vi "Pre Launch Init.vi"(11 "Study Actor in":refnum<class "Study Actor.lvclass">) -> (0 "error out":errorcluster, 3 "Study Actor out":refnum<class "Study Actor.lvclass">)   [LabVIEW 2023, in "HAL GOOP4.lvlib" / "Study Actor.lvlib" / "Study Actor.lvclass"]
doc: "Initializes the panel actor. Creates the Panel Helper.\n\n----\nPlease see the following web address for additional documentation and tutorial information:\nhttp://www.mooregoodideas.com/mgi-panel-manager/\n\nAuthor: Derek Trepanier\n\nCopyright (c) 2018, Moore Good Ideas, Inc.\n\nAll rights reserved.\n\nRedistribution and use in source and binary forms, with or without modification, are permitted provided that the following conditions are met:\n\n * Redistributions of source code must retain the above copyright notice, this list of conditions and the following disclaimer.\n * Redistributions in binary form must reproduce the above copyright notice, this list of conditions and the following disclaimer in the documentation and/or other materials provided with the distribution.\n * Neither the name of Moore Good Ideas, Inc. nor the names of its contributors may be used to endorse or promote products derived from this software without specific prior written permission.\n\nTHIS SOFTWARE IS PROVIDED BY THE COPYRIGHT HOLDERS AND CONTRIBUTORS \"AS IS\" AND ANY EXPRESS OR IMPLIED WARRANTIES, INCLUDING, BUT NOT LIMITED TO, THE IMPLIED WARRANTIES OF MERCHANTABILITY AND FITNESS FOR A PARTICULAR PURPOSE ARE DISCLAIMED. IN NO EVENT SHALL THE COPYRIGHT OWNER OR CONTRIBUTORS BE LIABLE FOR ANY DIRECT, INDIRECT, INCIDENTAL, SPECIAL, EXEMPLARY, OR CONSEQUENTIAL DAMAGES (INCLUDING, BUT NOT LIMITED TO, PROCUREMENT OF SUBSTITUTE GOODS OR SERVICES; LOSS OF USE, DATA, OR PROFITS; OR BUSINESS INTERRUPTION) HOWEVER CAUSED AND ON ANY THEORY OF LIABILITY, WHETHER IN CONTRACT, STRICT LIABILITY, OR TORT (INCLUDING NEGLIGENCE OR OTHERWISE) ARISING IN ANY WAY OUT OF THE USE OF THIS SOFTWARE, EVEN IF ADVISED OF THE POSSIBILITY OF SUCH DAMAGE."
uses:
  Study Actor.lvclass
  Study Actor.lvclass/Study Actor.ctl
  <vilib>/MGI/Panel Manager/Panel Actor/Panel Actor/Panel Actor.lvclass
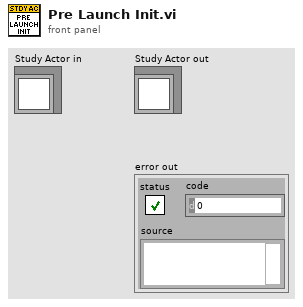
[diagram p1: front panel]
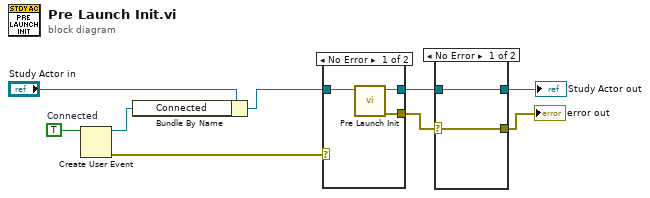
[diagram p0: block diagram]
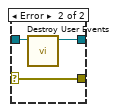
[diagram p2: hidden frame]
diagram:
  w9 = TRUE  # Connected
  n1 = Create User Event(user event datatype=w9) -> (user event=w7:refnum<user-event>, error out=w5:errorcluster)  [unwired: 1 in]
  n2 = Bundle By Name(cluster="Study Actor in", "Connected"=w7) -> (w6:refnum<class "Study Actor.lvclass">)
  n3 = case shown="No Error" w5 {
    selector: w5 -> [_ w13]
    tunnel: [w12 w13] -> w2
    tunnel: [w11 w14] -> w4
    tunnel: w6 -> [w10 w14]
    frame No Error {
      n4 = call-parent "Pre Launch Init.vi"("Panel Actor in"=w10) -> ("error out"=w12:errorcluster, "Panel Actor out"=w11:refnum<class "Study Actor.lvclass">)  [unwired: 9 in]
    }
    frame Error {
    }
  }
  n5 = case shown="No Error" w2 {
    selector: w2 -> [w16 w17]
    tunnel: w4 -> [w15 w19]
    tunnel: [w15 w18] -> w3
    tunnel: [w16 w17] -> w1
    frame No Error {
    }
    frame Error {
      n6 = call "Destroy User Events.vi"("Study Actor in"=w19) -> ("Study Actor out"=w18:refnum<class "Study Actor.lvclass">)  [unwired: 10 in]
    }
  }
  "error out" <- w1
  "Study Actor out" <- w3
